vi "AssertDisabled.vi"(0 "VI Reference In":refnum<vi>, 1 "Test Label":string, 2 "delimiter (>>)":string=">>", 3 "Assert Only? (F)":bool, 5 "Control Path":string, 11 "Error In":errorcluster, 12 "Assert Interval(10 ms)":u32=10, 13 "Timeout(5 sec)":dbl=5.0) -> (4 "VI Reference Out":refnum<vi>, 6 "Test Control State":T1(ring), 15 "Error Out":errorcluster)   [LabVIEW 2016, in "Drona.lvlib" / "AssertControlDisable.lvlib"]
doc: "Asserts if the control is disabled.\n\nThe input control name is given as a string , incase of path, use delimiters inbetween the path.\nThis VI checks until the control is disabled."
uses:
  AssertControlDisable.lvlib
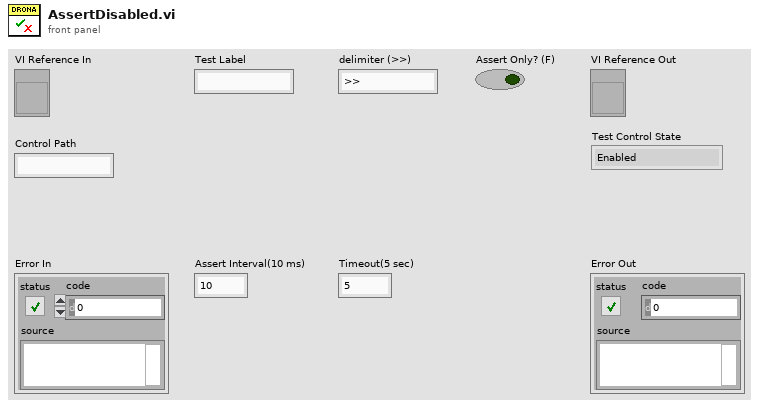
[diagram p1: front panel]
types:
  T1 = enum8{"Enabled", "Disabled", "Disabled and Grayed Out"}
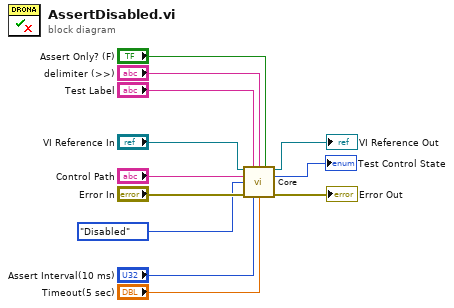
[diagram p0: block diagram]
diagram:
  n1 = call "Core.vi"("VI Reference In"="VI Reference In", "Label"="Test Label", "delimiter (>>)"="delimiter (>>)", "Assert Only? (F)"="Assert Only? (F)", "Control Path"="Control Path", "Disabled"=T1."Disabled", "Error In"="Error In", "Assert Interval(10 ms)"="Assert Interval(10 ms)", "Timeout(5 sec)"="Timeout(5 sec)") -> ("VI Reference Out"=→"VI Reference Out":refnum<vi>, "Test Control State"=→"Test Control State":T1, "Error Out"=→"Error Out":errorcluster)  [unwired: 4 in]
